vi "Grid_Finish.vi"(7 "Part of multigrid":bool, 8 "Error in":errorcluster, 9 "FileRefs":T2, 10 "Settings":T1={"Drift Correction Settings"={"Drift Correction every"=80, "Drift correction Pixels"=256, "Channel index (0-23)"=0, "MaxImagesBack"=2, "Threshold"=2, "Increment"=8, "max applied Drift Correction"=20, "Correct Drift"=TRUE, "Correlate"=0, "Correct z drift"=FALSE, "zdrift \nDuration (s)"=0.0}, "Spectroscopy Setting"={"Imaging Current"=1e-11, "ref Current"=7e-11, "tip Speed (m/s)"=2e-09, "Imaging Bias"=0.02, "ref Bias"=-0.1, "preSTS delay [ms]"=500, "STS z offset"=2e-10, "during Spec Bias (V)"=-0.1, "trigger1 < Hz"=0.0, "trigger 2 >Hz"=0.0, "autoStop"=FALSE, "Spectroscopy"=0, "PLL ON/OFF"=TRUE, "readjust setpoint every "=1, "z Reference"=FALSE, "Lock In"=TRUE}, "Misc"={"File name"="symmetric_node_zOff=200p", "Email when finished"="cornelius.krull@monash.edu,Dhaneesh.Gopalakrishnan@monash.edu,marina.castelli@monash.edu"}, "Grid Settings"={"type"=1, "type order"=1, "X pixel"=0, "Y pixel"=0, "Grid_Parms"={"center X (m)"=0.0, "center Y (m)"=0.0, "width (m)"=0.0, "height (m)"=0.0, "angle (deg)"=0.0}}} {"Grid Settings"."type order" items=["Grid", "Random", "Adam7"]; "Grid Settings"."type" items=["Line", "Grid"]; "Spectroscopy Setting"."Spectroscopy" items=["Bias", "zSpec"]; "Spectroscopy Setting"."trigger 2 >Hz" format="%#_6p"; "Spectroscopy Setting"."trigger1 < Hz" format="%#_6p"; "Spectroscopy Setting"."during Spec Bias (V)" format="%#_5p"; "Spectroscopy Setting"."STS z offset" format="%#_6p"; "Spectroscopy Setting"."ref Bias" format="%#_6p"; "Spectroscopy Setting"."Imaging Bias" format="%#_6p"; "Spectroscopy Setting"."tip Speed (m/s)" format="%.2p"; "Spectroscopy Setting"."ref Current" format="%#_6p"; "Spectroscopy Setting"."Imaging Current" format="%#_6p"; "Drift Correction Settings"."Correlate" items=["first Frame", "successive Frames"]; "Drift Correction Settings"."max applied Drift Correction" min=1 max=100 step=1 format="%.0p"; "Drift Correction Settings"."Threshold" min=1 step=1; "Drift Correction Settings"."Channel index (0-23)" items=["Current"=0, "Z (m)"=14]}, 11 "Application reference":refnum<vi>) -> ()   [LabVIEW 2014]
uses:
  <userlib>/Nanonis Prog Interface V5/Nanonis Prog Interface.lvlib
panel:
  # "z Spectroscopy"
  # "GRID points"
  # "Increase this if no Drift was detected for \na certain number of images"
  # "% of image size"
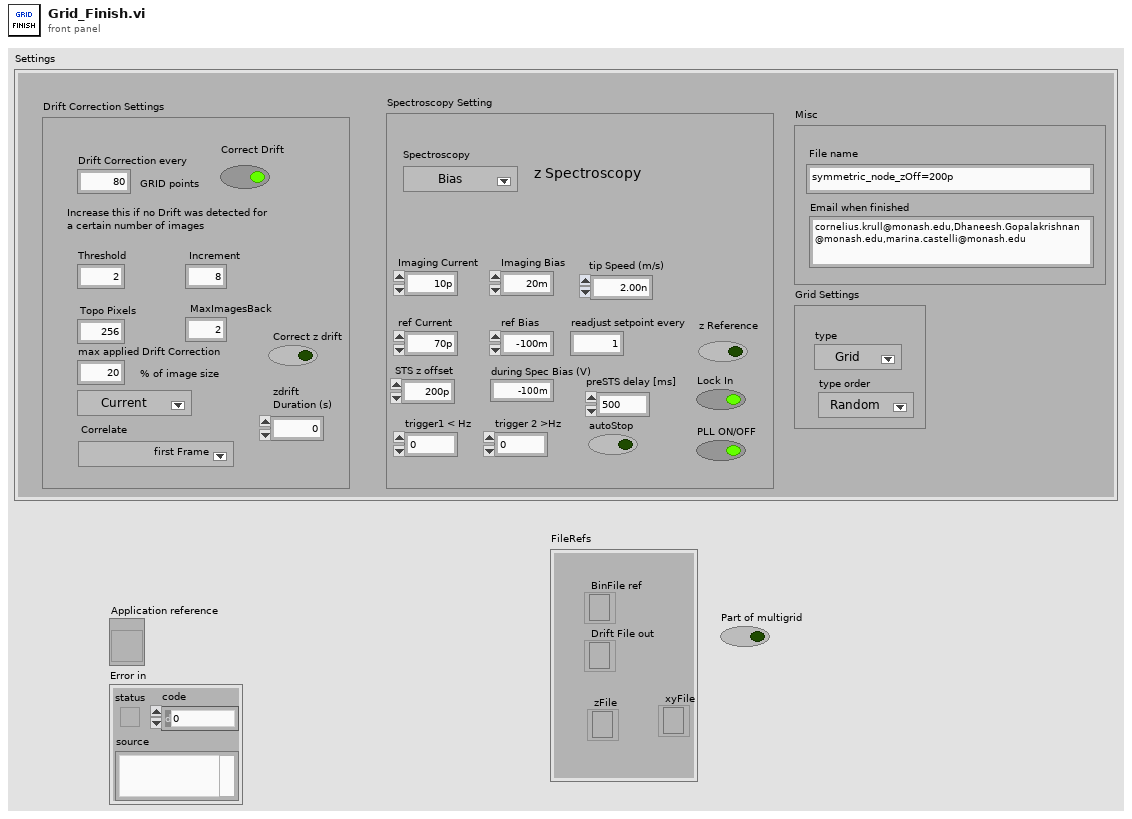
[diagram p1: front panel]
types:
  T1 = cluster{"Drift Correction Settings":cluster{"Drift Correction every":i32, "Drift correction Pixels":i32, "Channel index (0-23)":u8, "MaxImagesBack":i32, "Threshold":i32, "Increment":i32, "max applied Drift Correction":i32, "Correct Drift":bool, "Correlate":u16, "Correct z drift":bool, "zdrift \nDuration (s)":dbl}, "Spectroscopy Setting":cluster{"Imaging Current":dbl, "ref Current":dbl, "tip Speed (m/s)":sgl, "Imaging Bias":dbl, "ref Bias":dbl, "preSTS delay [ms]":u32, "STS z offset":dbl, "during Spec Bias (V)":sgl, "trigger1 < Hz":sgl, "trigger 2 >Hz":sgl, "autoStop":bool, "Spectroscopy":u16, "PLL ON/OFF":bool, "readjust setpoint every ":i32, "z Reference":bool, "Lock In":bool}, "Misc":cluster{"File name":string, "Email when finished":string}, "Grid Settings":cluster{"type":u16, "type order":u16, "X pixel":i32, "Y pixel":i32, "Grid_Parms":cluster{"center X (m)":sgl, "center Y (m)":sgl, "width (m)":sgl, "height (m)":sgl, "angle (deg)":sgl}}}
  T2 = cluster{"Drift File out":refnum<file>, "zFile":refnum<file>, "BinFile ref":refnum<file>, "xyFile":refnum<file>}
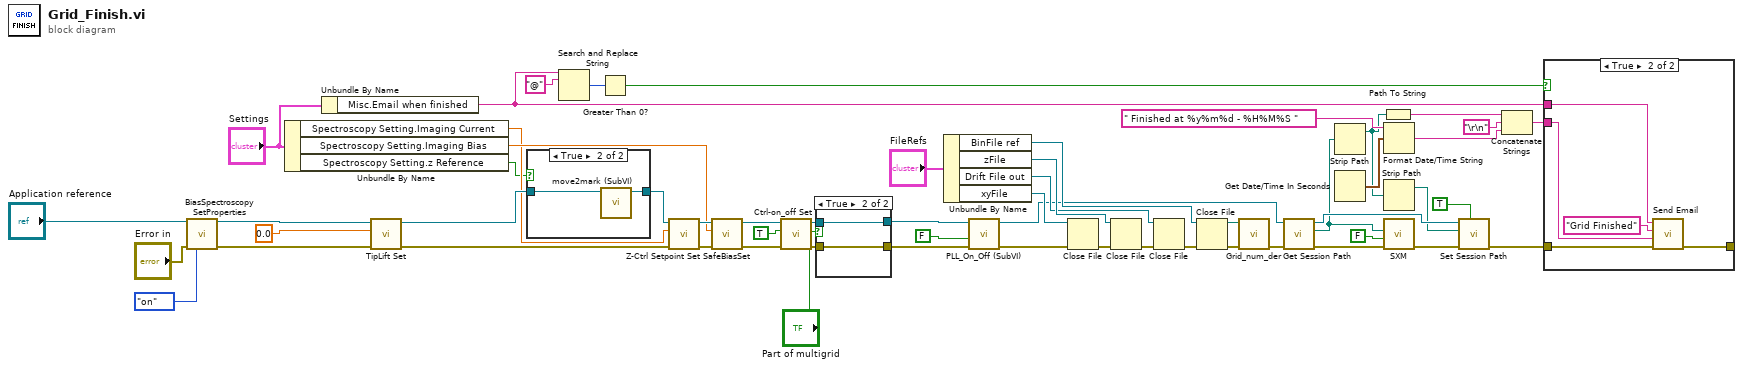
[diagram p0: block diagram]
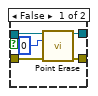
[diagram p2: hidden frame]
diagram:
  n1 = call <userlib>:"BiasSpectroscopy SetProperties.vi"("Application ref in"="Application reference", "Error in (no error)"="Error in", "Z-Controller hold (no change)"=enum16{"no change", "on", "off"}."on") -> ("Application ref out"=w45:refnum<vi>, "Error out"=w15:errorcluster)  [unwired: 11 in]
  n2 = Unbundle By Name("Settings") -> ("Spectroscopy Setting.Imaging Current"=w11:dbl, "Spectroscopy Setting.Imaging Bias"=w12:dbl, "Spectroscopy Setting.z Reference"=w2:bool)
  n3 = Unbundle By Name("Settings") -> ("Misc.Email when finished"=w28:string)
  n4 = call <userlib>:"TipLift Set.vi"("error in (no error)"=w15, "TipLift (m)"=sgl 0.0, "Application ref in"=w45) -> ("error out"=w14:errorcluster, "Application ref out"=w43:refnum<vi>)  [unwired: 7 in]
  n5 = case shown="True" w2 {
    tunnel: w43 -> [w57 w59]
    tunnel: [w57 w58] -> w34
    frame False {
    }
    frame True {
      n6 = call "move2mark (SubVI).vi"("Application in"=w59) -> ("Application out"=w58:refnum<vi>)  [unwired: 10 in]
    }
  }
  n7 = Search and Replace String(input string=w28, search string="@") -> (number of replacements=w48:i32)  [unwired: 6 in, 3 out]
  n8 = Greater Than 0?(x=w48) -> (x > 0?=w47:bool)
  n9 = call <userlib>:"Z-Ctrl Setpoint Set.vi"("error in (no error)"=w14, "Z Controller setpoint"=w11, "Application ref in"=w34) -> ("error out"=w13:errorcluster, "Application ref out"=w33:refnum<vi>)  [unwired: 7 in]
  n10 = call "SafeBiasSet.vi"("Application ref in"=w33, "Bias (V)"=w12, "error in (no error)"=w13) -> ("Application ref out"=w40:refnum<vi>, "Error out"=w37:errorcluster)  [unwired: 6 in]
  n11 = call <userlib>:"Ctrl-on_off Set.vi"("error in (no error)"=w37, "Z Controller ON/OFF"=TRUE, "Application ref in"=w40) -> ("error out"=w36:errorcluster, "Application ref out"=w42:refnum<vi>)  [unwired: 7 in]
  n12 = case shown="True" "Part of multigrid" {
    tunnel: w42 -> [w63 w66]
    tunnel: [w62 w66] -> w39
    tunnel: w36 -> [w61 w65]
    tunnel: [w60 w65] -> w35
    frame False {
      n13 = call <userlib>:"Point Erase.vi"("Application ref in"=w63, "Point index (-1=All points)"=0, "error in (no error)"=w61) -> ("Application ref out"=w62:refnum<vi>, "error out"=w60:errorcluster)  [unwired: 11 in]
    }
    frame True {
    }
  }
  n14 = Unbundle By Name("FileRefs") -> ("BinFile ref"=w20:refnum<file>, "zFile"=w26:refnum<file>, "Drift File out"=w24:refnum<file>, "xyFile"=w9:refnum<file>)
  n15 = call "PLL_On_Off (SubVI).vi"("error in (no error)"=w35, "Output ON/OFF (F=OFF)"=FALSE, "Application in"=w39) -> ("error out"=w3:errorcluster, "Application out"=w5:refnum<vi>)  [unwired: 7 in]
  n16 = Close File(refnum=w9, error in=w3) -> (error out=w8:errorcluster)  [unwired: 1 out]
  n17 = Close File(refnum=w26, error in=w8) -> (error out=w25:errorcluster)  [unwired: 1 out]
  n18 = Close File(refnum=w24, error in=w25) -> (error out=w22:errorcluster)  [unwired: 1 out]
  n19 = Close File(refnum=w20, error in=w22) -> (path=w23:path, error out=w21:errorcluster)
  n20 = call "Grid_num_der.vi"("error in (no error)"=w21, "Binary Spectroscopy File"=w23) -> ("error out"=w19:errorcluster)  [unwired: 9 in]
  n21 = call <userlib>:"Get Session Path.vi"("error in (no error)"=w19, "Application ref in"=w5) -> ("error out"=w55:errorcluster, "Session path"=w18:path, "Application ref out"=w30:refnum<vi>)  [unwired: 7 in]
  n22 = Strip Path(path=w18) -> (stripped path=w10:path)  [unwired: 1 out]
  n23 = Get Date/Time In Seconds() -> (seconds since 1Jan1904=w29:timestamp)
  n24 = Path To String(path=w10) -> (string=w54:string)
  n25 = Format Date/Time String(time format string (%c)=" Finished at %y%m%d - %H%M%S ", seconds (now)=w29) -> (date/time string=w51:string)  [unwired: 1 in]
  n26 = Strip Path(path=w10) -> (stripped path=w17:path)  [unwired: 1 out]
  n27 = call "SXM.vi"("Path"=w18, "Delete"=FALSE, "error in"=w55) -> ("error out"=w31:errorcluster)  [unwired: 7 in]
  n28 = call <userlib>:"Set Session Path.vi"("Save settings to previous? (False)"=TRUE, "error in (no error)"=w31, "Session Folder"=w17, "Application ref in"=w30) -> ("error out"=w16:errorcluster)  [unwired: 6 in, 1 out]
  n29 = Concatenate Strings(w54, "\r\n", w51) -> (w53:string)
  n30 = case shown="True" w47 {
    tunnel: w16 -> [w67 w72]
    tunnel: w53 -> [_ w70]
    tunnel: w28 -> [_ w69]
    tunnel: [w67 w68] -> _
    frame False {
    }
    frame True {
      n31 = call "Send Email"("error in"=w72, "Message"=w70, "Subject"="Grid Finished", "Recipients"=w69) -> ("error out"=w68:errorcluster)  [unwired: 7 in]
    }
  }
